vi "Copy File to Directories.vi"(8 "error in (no error)":errorcluster, 10 "File to Deploy":path, 11 "Paths in":path[](array[path])) -> (0 "error out":errorcluster, 3 "Paths out":path[](array[path]))   [LabVIEW 2017]
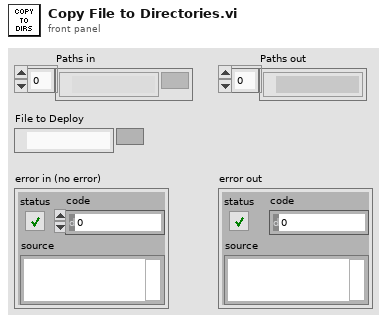
[diagram p1: front panel]
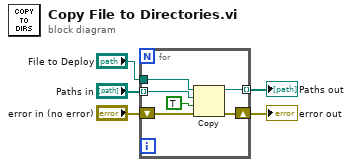
[diagram p0: block diagram]
diagram:
  n1 = for {
    tunnel: "Paths in" -> [w11] mode=indexing
    tunnel: "File to Deploy" -> [w10]
    shift-right: [w8] -> w5
    shift-left: "error in (no error)" -> [w9]
    tunnel: [w7] -> w4 mode=indexing
    n2 = Copy(8:w9, 9:TRUE ("overwrite (F)"), 10:w11, 11:w10) -> (0:w8:errorcluster, 3:w7:path)  [unwired: 1 in, 1 out]
  }
  "error out" <- w5
  "Paths out" <- w4
